vi "Setup subWorkers.vi"(8 "error in":errorcluster, 11 "UI Cam Basler in":refnum<class "UI Cam Basler.lvclass">) -> (0 "error out":errorcluster, 3 "UI Cam Basler out":refnum<class "UI Cam Basler.lvclass">)   [LabVIEW 2023, in "UI Cam Basler.lvclass"]
doc: "<b>Note: Do not change the code in this VI!</b>\nThis VI performs a setup of all the statically-linked subWorkers that belong to the Worker that calls this VI. This VI is created automatically by the 'Create/Add Worker' tool and must be called <b>before</b> any statically linked subWorkers are called."
uses:
  UI Cam Basler.lvclass
  UI Cam Basler.lvclass/UI Cam Basler.ctl
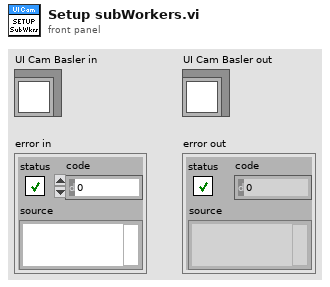
[diagram p1: front panel]
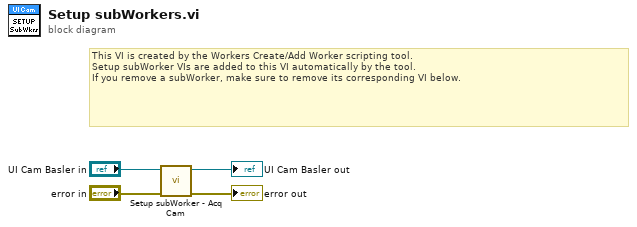
[diagram p0: block diagram]
diagram:
  # "This VI is created by the Workers Create/Add Worker scripting tool.\nSetup subWorker VIs are added to this VI automatically by the tool.\nIf you remove a subWorker, make sure to remove its corresponding VI below."
  n1 = call "Setup subWorker - Acq Cam.vi"("error in"="error in", "UI Cam Basler in"="UI Cam Basler in") -> ("error out"=→"error out":errorcluster, "UI Cam Basler out"=→"UI Cam Basler out":refnum<class "UI Cam Basler.lvclass">)  [unwired: 8 in]
